vi "Execute_Y2_Measure.vi"(0 "VISA In":refnum<visa-resource-name>, 1 "Y2 axis settings":T1, 2 "X-Axis Trace":dbl[](array[numeric]), 3 "error in (no error)":errorcluster, 4 "Y2 axis on/off":bool) -> (8 "Y2 Output Cluster":cluster{"trace":dbl[], "trace":dbl[]}, 10 "error out":errorcluster)   [LabVIEW 2012]
panel:
  out "VISA Out":refnum<visa-resource-name>
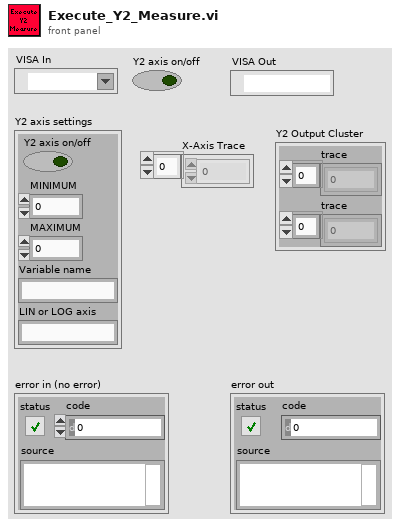
[diagram p1: front panel]
types:
  T1 = cluster{"Y2 axis on/off":bool, "MINIMUM":ext, "MAXIMUM":ext, "Variable name":string, "LIN or LOG axis":string}
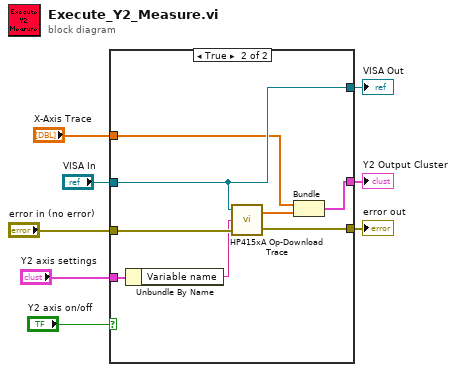
[diagram p0: block diagram]
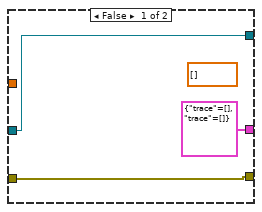
[diagram p2: hidden frame]
diagram:
  n1 = case shown="True" "Y2 axis on/off" {
    tunnel: "error in (no error)" -> [w11 w19]
    tunnel: "VISA In" -> [w9 w13]
    tunnel: [w11 w18] -> w4
    tunnel: [cluster{"trace":dbl[], "trace":dbl[]} {"trace"=[], "trace"=[]} w16] -> w8
    tunnel: "Y2 axis settings" -> [_ w15]
    tunnel: [w9 w13] -> w2
    tunnel: "X-Axis Trace" -> [_ w12]
    frame False {
      (unwired) dbl[] [] ("trace")
    }
    frame True {
      n2 = Unbundle By Name(w15) -> ("Variable name"=w14:string)
      n3 = call "HP415xA Op-Download Trace.vi"("error in (no error)"=w19, "trace (variable) name"=w14, "VISA session"=w13) -> ("error out"=w18:errorcluster, "trace"=w17:dbl[])
      n4 = Bundle("X-Axis Trace"=w12, "trace"=w17) -> (w16:cluster{"X-Axis Trace":dbl[], "trace":dbl[]})  [unwired: 1 in]
    }
  }
  "Y2 Output Cluster" <- w8
  "error out" <- w4
  "VISA Out" <- w2
